vi "Initialize.vi"(7 "ChannelName":string="Setpoint.ch%d.SP", 8 "error in":errorcluster, 9 "Number of Channels":u32=1, 10 "Instance Name":string, 11 "OnOff in":refnum<class "OnOff.lvclass">) -> (0 "error out":errorcluster, 3 "OnOff out":refnum<class "OnOff.lvclass">)   [LabVIEW 2023, in "OnOff.lvclass"]
uses:
  OnOff.lvclass
  OnOff.lvclass/OnOff.ctl
  <vilib>/ADAS Replay HIL/Channels/Tag Wrapper/Polymorphic/Open Producer Tag (I32).vi/45cd6eaa-a1ce-41a4-8aba-62a49d103d7e.vi
  <vilib>/ADAS Replay HIL/Channels/Tag Wrapper/Polymorphic/Set Default Value (I32).vi/228e99de-6fcf-414d-86fc-dc277c7b351f.vi
  <vilib>/ADAS Replay HIL/Channels/Tag Wrapper/Polymorphic/Open Consumer Tag (Boolean).vi/bacb721e-673a-491a-accd-959f2e1f334e.vi
  <vilib>/ADAS Replay HIL/Channels/Tag Wrapper/Polymorphic/Set Default Value (Boolean).vi/228e99de-6fcf-414d-86fc-dc277c7b351f.vi
  <vilib>/ADAS Replay HIL/Channels/Tag Wrapper/Polymorphic/Open Producer Tag (I32).vi/45cd6eaa-a1ce-41a4-8aba-62a49d103d7e.vi/c28b0ead-42ad-4072-80a2-aca7f2bd7ce3.vi
  <vilib>/ADAS Replay HIL/Channels/Tag Wrapper/Polymorphic/Set Default Value (I32).vi/228e99de-6fcf-414d-86fc-dc277c7b351f.vi/4bc1c15b-36ab-481f-b8dd-c64075ce723a.vi
  <vilib>/ADAS Replay HIL/Channels/Tag Wrapper/Polymorphic/Open Consumer Tag (Boolean).vi/bacb721e-673a-491a-accd-959f2e1f334e.vi/c28b0ead-42ad-4072-80a2-aca7f2bd7ce3.vi
  <vilib>/ADAS Replay HIL/Channels/Tag Wrapper/Polymorphic/Set Default Value (Boolean).vi/228e99de-6fcf-414d-86fc-dc277c7b351f.vi/4bc1c15b-36ab-481f-b8dd-c64075ce723a.vi
  <vilib>/ADAS Replay HIL/AdasHilServices/AdasHilServices Fill In Error Info Ex.vi
  <vilib>/ADAS Replay HIL/Channels/Tag Wrapper/Polymorphic/Open Consumer Tag (Boolean).vi
  <vilib>/ADAS Replay HIL/Channels/Tag Wrapper/Polymorphic/Set Default Value (I32).vi
  <vilib>/ADAS Replay HIL/Channels/Tag Wrapper/Polymorphic/Open Producer Tag (I32).vi
  <vilib>/ADAS Replay HIL/Channels/Tag Wrapper/Polymorphic/Set Default Value (Boolean).vi
  Utilities/Utilities.lvlib
  <vilib>/ADAS Replay HIL/Channels/Tag Wrapper/Tag Wrapper.lvlib
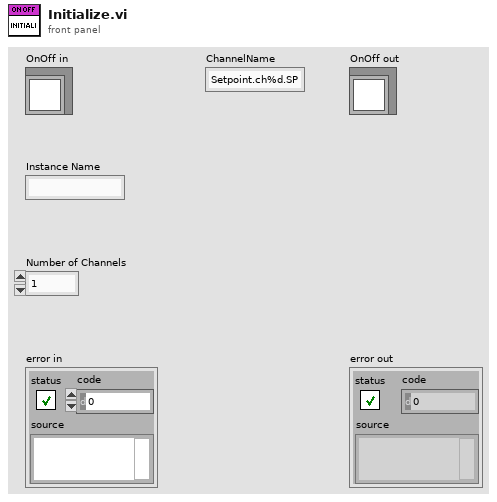
[diagram p1: front panel]
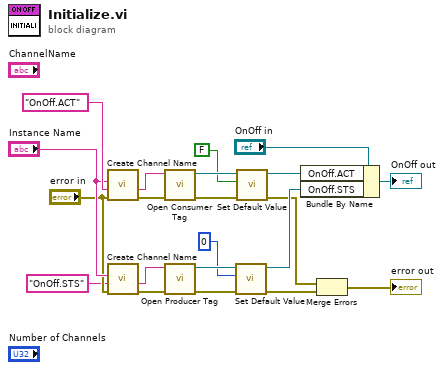
[diagram p0: block diagram]
diagram:
  n1 = call "Create Channel Name.vi"("error in"="error in", "Channel Name"="OnOff.ACT", "Plugin Name"="Instance Name") -> ("error out"=w21:errorcluster, "Data Channel Name"=w19:string)  [unwired: 7 in]
  n2 = call "Create Channel Name.vi"("error in"="error in", "Channel Name"="OnOff.STS" ("ChannelName"), "Plugin Name"="Instance Name") -> ("error out"=w11:errorcluster, "Data Channel Name"=w9:string)  [unwired: 7 in]
  n3 = call-poly <vilib>:"Open Consumer Tag.vi"("error in"=w21, "Channel Name"=w19) -> ("error out"=w20:errorcluster, "ADAS HIL Channel"=w18:refnum<k21>)  [unwired: 8 in]
  n4 = call-poly <vilib>:"Open Producer Tag.vi"("error in"=w11, "Channel Name"=w9) -> ("error out"=w10:errorcluster, "ADAS HIL Channel"=w12:refnum<k21>)  [unwired: 8 in]
  n5 = call-poly <vilib>:"Set Default Value.vi"("error in"=w10, "Default Value"=0, "ADAS HIL Channel in"=w12) -> ("error out"=w13:errorcluster, "ADAS HIL Channel out"=w15:refnum<k21>)  [unwired: 7 in]
  n6 = call-poly <vilib>:"Set Default Value.vi"("error in"=w20, "Default Value"=FALSE, "ADAS HIL Channel in"=w18) -> ("error out"=w14:errorcluster, "ADAS HIL Channel out"=w16:refnum<k21>)  [unwired: 7 in]
  n7 = Bundle By Name(cluster="OnOff in", "OnOff.ACT"=w16, "OnOff.STS"=w15) -> (→"OnOff out":refnum<class "OnOff.lvclass">)
  n8 = Merge Errors(w14, w13) -> (→"error out":errorcluster)
